vi "Compute.vi"(8 "error in (no error)":errorcluster, 9 "Data Channels":T4, 10 "x-var":T1, 11 "Multiply in":refnum<class "Multiply.lvclass">) -> (0 "error out":errorcluster, 1 "Add'l Data Channels":T4, 3 "Multiply out":refnum<class "Multiply.lvclass">)   [LabVIEW 2012, in "Multiply.lvclass"]
doc: "Given a data channel and an x-coordinate, compute and return one or more new data channels."
uses:
  Multiply.lvclass
  Instruments/Utility Classes/Readable/Data Channels.ctl
  Instruments/Utility Classes/Readable/Data Channel.ctl
  Instruments/Utility Classes/Readable/Data Point.ctl
  Instruments/Utility Classes/Readable/Time.ctl
  Instruments/Utility Classes/Readable/X.ctl
  Multiply.lvclass/Multiply.ctl
  Instruments/Utility Classes/Readable/Readable.lvclass
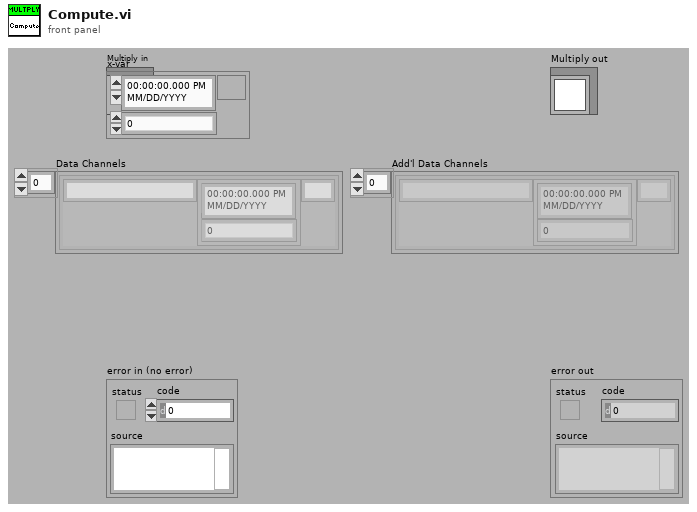
[diagram p1: front panel]
types:
  T1 = typedef "Readable.lvclass/Data Point.ctl" = cluster{"t":T2, "x":T3}
  T2 = typedef "Readable.lvclass/Time.ctl" = timestamp
  T3 = typedef "Readable.lvclass/X.ctl" = dbl
  T4 = typedef "Readable.lvclass/Data Channels.ctl" = T5[]
  T5 = typedef "Readable.lvclass/Data Channel.ctl" = cluster{"Name":string, "Data Point":T1, "Unit":string}
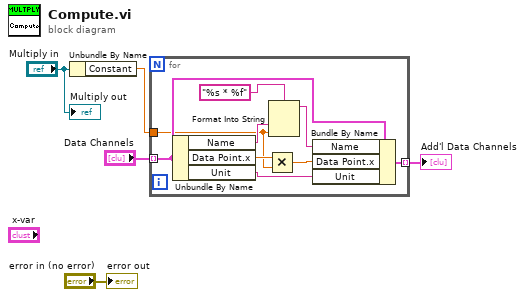
[diagram p0: block diagram]
diagram:
  n1 = Unbundle By Name("Multiply in") -> ("Constant"=w2:dbl)
  n2 = for {
    tunnel: "Data Channels" -> [w12] mode=indexing
    tunnel: [w7] -> w3 mode=indexing
    tunnel: w2 -> [w6]
    n3 = Unbundle By Name(w12) -> ("Name"=w13:string, "Data Point.x"=w10:T3, "Unit"=w8:string)
    n4 = Multiply(x=w10, y=w6) -> (x*y=w9:T3)
    n5 = Format Into String(format string="%s * %f", w13, w6) -> (resulting string=w11:string)  [unwired: 2 in, 1 out]
    n6 = Bundle By Name(cluster=w12, "Name"=w11, "Data Point.x"=w9, "Unit"=w8) -> (w7:T5)
  }
  "Add'l Data Channels" <- w3
  "error out" <- "error in (no error)"
  "Multiply out" <- "Multiply in"
